vi "Folder.vi"(11 "Folders":T1) -> (2 "found?":bool, 3 "FolderPath":path, 5 "Folder name":string)   [LabVIEW 2015, in "Design Server.lvlib"]
uses:
  Design Server.lvlib
  Folders.ctl
  <vilib>/Utility/config.llb/Read Key (Path).vi
  <vilib>/Utility/config.llb/NI_LVConfig.lvlib
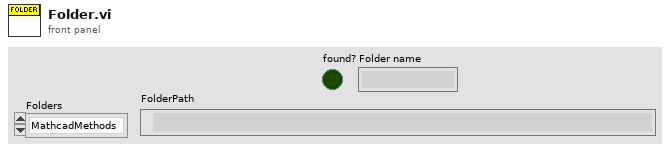
[diagram p1: front panel]
types:
  T1 = typedef "Design Server.lvlib/Folders.ctl" = enum16{"MathcadMethods", "RequestedDesigns", "CompletedDesigns", "MathcadCode", "CollabnetSVN.exe"}
  T2 = typedef "NI_LVConfig.lvlib/Config Data RefNum.ctl" = refnum<k1>
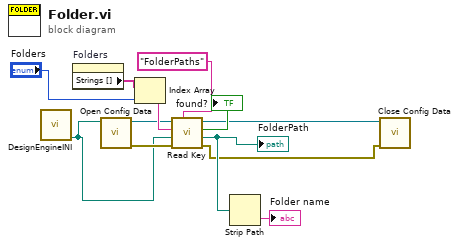
[diagram p0: block diagram]
diagram:
  n1 = call "DesignEngineINI.vi"() -> ("Ini file path"=w7:path)  [unwired: 6 in, 1 out]
  n2 = property on="Folders" class="Enum (strict)"() -> ("Strings []"=w11:string[])  [unwired: 2 in, 2 out]
  n3 = call <vilib>:"Open Config Data.vi"("configuration file path"=w7) -> ("error out"=w12:errorcluster, "refnum"=w6:T2)  [unwired: 8 in, 1 out]
  n4 = Index Array(array=w11, index="Folders") -> (element=w9:string)
  n5 = call-poly <vilib>:"Read Key.vi"("section"="FolderPaths", "error in (no error)"=w12, "default value"=w7, "key"=w9, "refnum"=w6) -> ("error out"=w1:errorcluster, "value"=w4:path, "found?"=→"found?":bool, "refnum out"=w2:T2)  [unwired: 3 in]
  "FolderPath" <- w4
  n6 = Strip Path(path=w4) -> (name=→"Folder name":string)  [unwired: 1 out]
  n7 = call <vilib>:"Close Config Data.vi"("error in (no error)"=w1, "refnum"=w2) -> ()  [unwired: 8 in, 2 out]
